vi "STANDALONE_VI.vi"() -> ()   [LabVIEW 2018]
uses:
  <vilib>/Instr/_visa.llb/VISA Open Access Mode.ctl
  <vilib>/express/express signal manip/GetorSetDDTAttributes/Shared VIs/TimeType.ctl
  <vilib>/Analysis/baseanly.llb/Mean (DBL).vi
  <vilib>/Analysis/2dsp.llb/1D Auto Correlation (DBL).vi
  <vilib>/Instr/_visa.llb/VISA Configure Serial Port (Instr).vi
  <vilib>/express/express signal manip/GetorSetDDTAttributes/Shared VIs/TimeMode Enum to Boolean.vi
  <vilib>/express/express shared/transition.llb/Dynamic To Waveform Array.vi
  <vilib>/express/express signal manip/GetorSetDDTAttributes/Set DDT Attributes/SetT0.vi
  <vilib>/express/express shared/transition.llb/Waveform Array To Dynamic.vi
  <vilib>/Analysis/2dsp.llb/1D Cross Correlation (DBL).vi
  <vilib>/express/express signal manip/GetorSetDDTAttributes/Set DDT Attributes/Set DDT Properties.xnode
  <vilib>/express/express signal manip/GetorSetDDTAttributes/Shared VIs/GetSetShared.lvlib
  <vilib>/Analysis/NI_AALPro.lvlib
  <vilib>/Analysis/NI_AALBase.lvlib
panel:
  out "DEBUG BUFFER":string
  out "Load Force (N)":dbl
  out "Grip Force (N)":dbl
  out "Calibration Complete":bool
  in  "?":bool
  out "x .or. y? 2":bool
  out "Load Force Plot":dynamicdata(graph)
  out "Grip Force Plot":dynamicdata(graph)
  out "x-y 4":u32
  out "Goniometer Angle Plot":dynamicdata(graph)
  out "Elbow Angle (deg)":dbl
  in  "Start Training\nButton":bool
  out "Calibration Timer":string caption="Elapsed Time Text"
  out "Elbow Angle Offset":dbl format="%0.2f"
  out "Grip Force at MZ":dbl format="%0.2f"
  out "Load Force at MZ":dbl format="%0.2f"
  in  "Calibrate System\nButton":bool
  in  "VISA resource name":refnum<visa-resource-name>="COM4"
  out "error out":errorcluster
  out "x*y":dbl
  out "max index(es)":i32
  out "max":dbl
  out "max value":dbl
  out "size":i32
  out "Waveform Graph":dbl[](graph)
  out "max index":i32
  out "Delay (ms)":i32
  out "GF min":dbl
  out "GF max":dbl
  out "LF min":dbl
  out "LF max":dbl
  # "SET UP"
  # "PLOTS"
  # "TRAINING SESSION"
  # "SYSTEM CALIBRATION"
  # "REAL-TIME DATA"
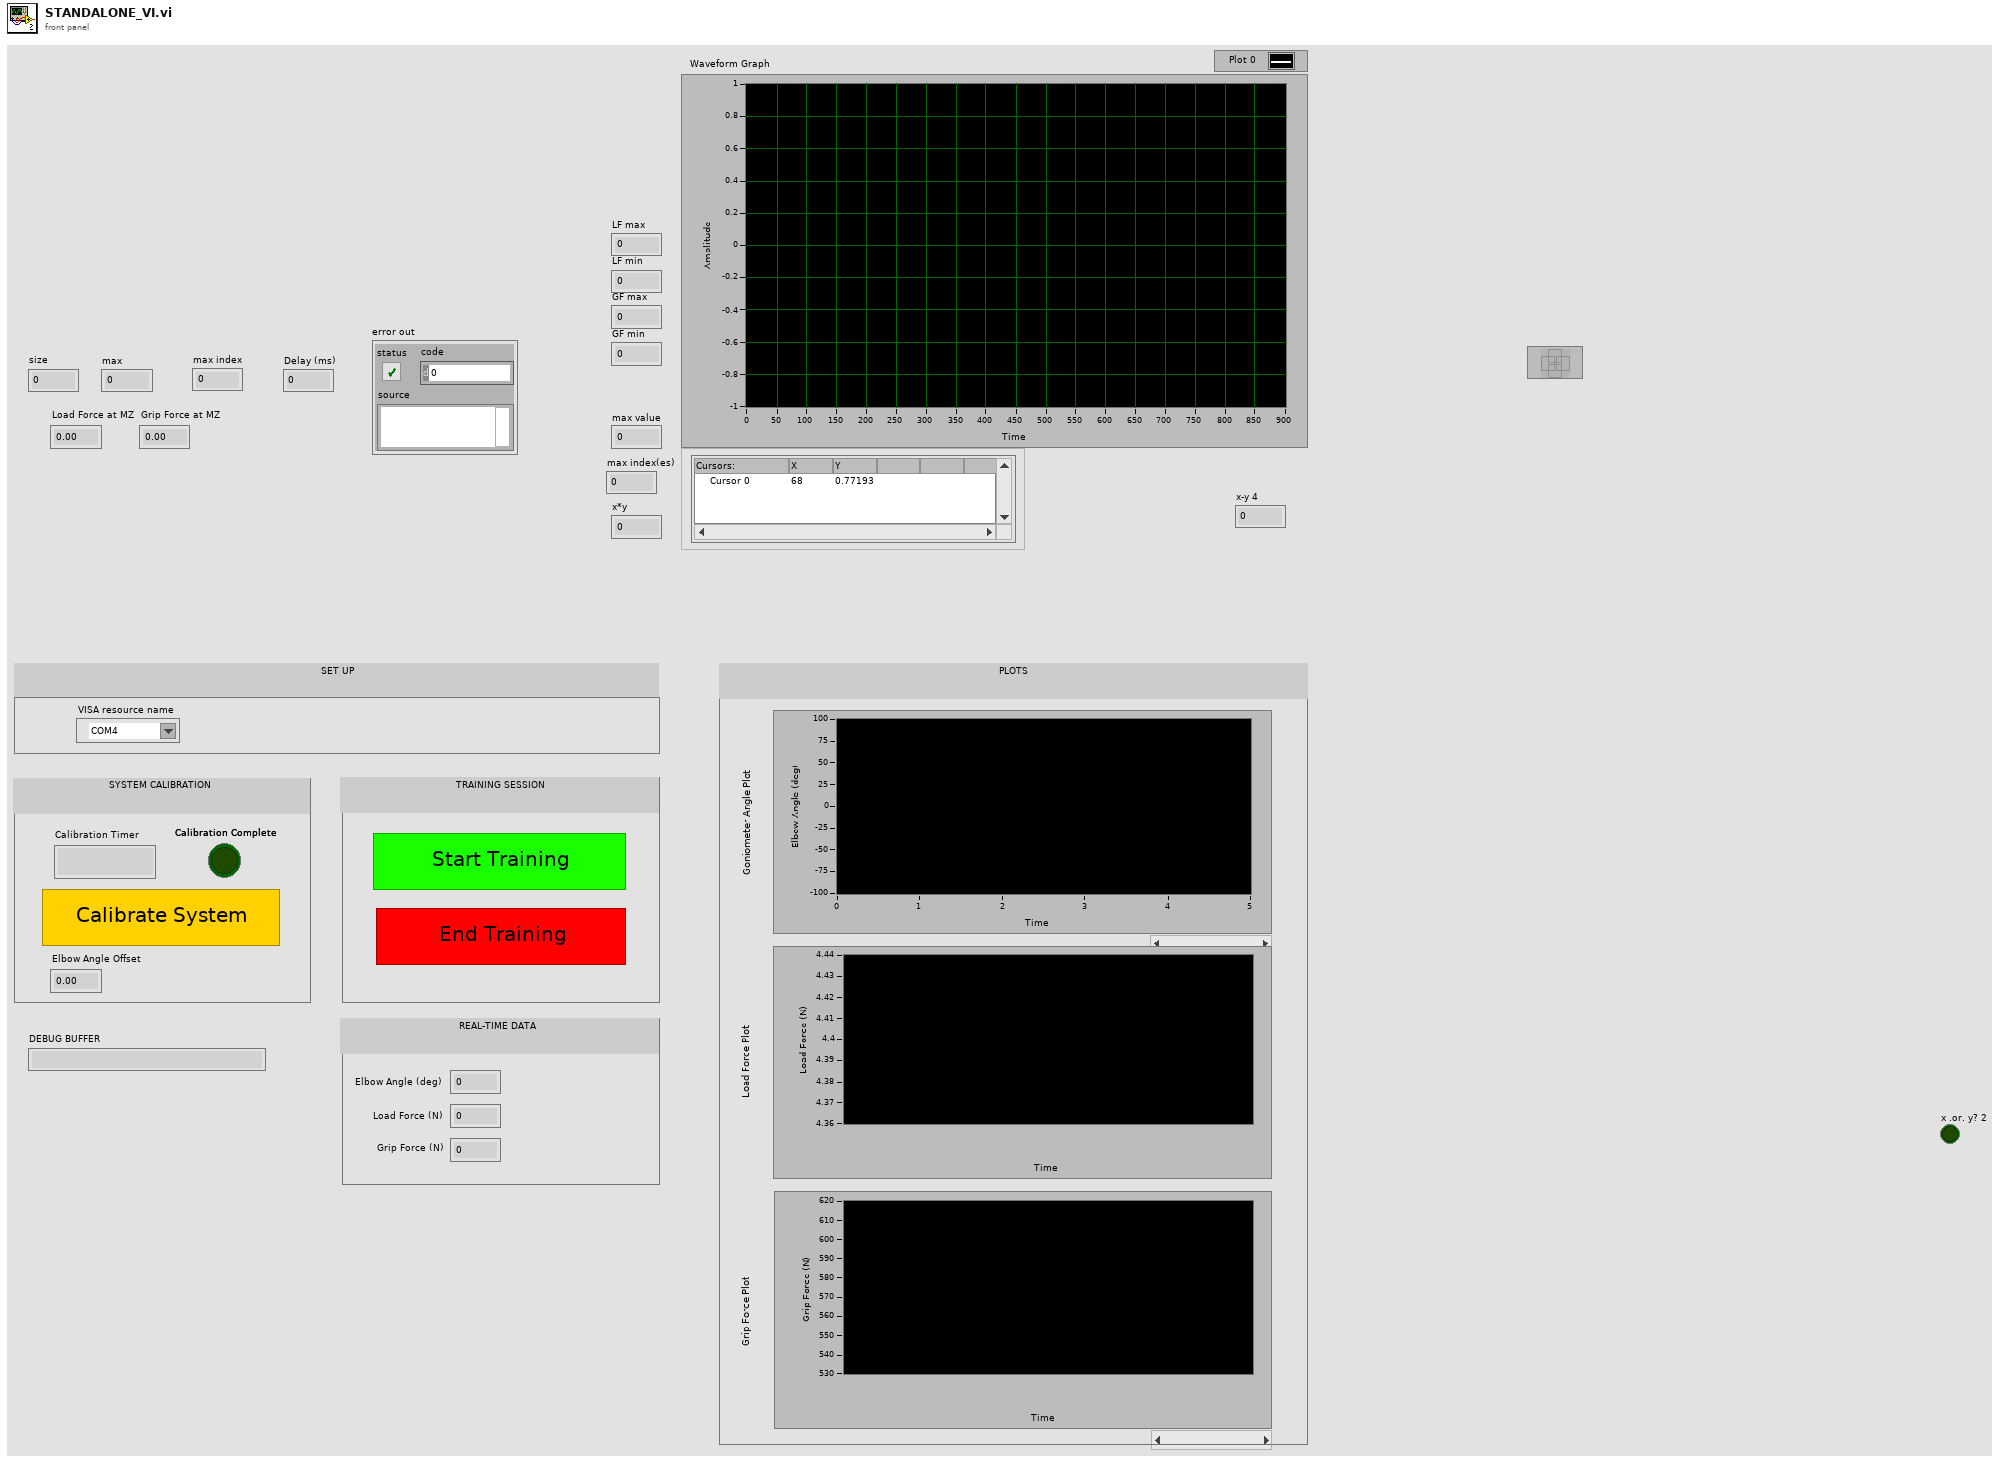
[diagram p1: front panel]
types:
  T1 = typedef "VISA Open Access Mode.ctl" = u32
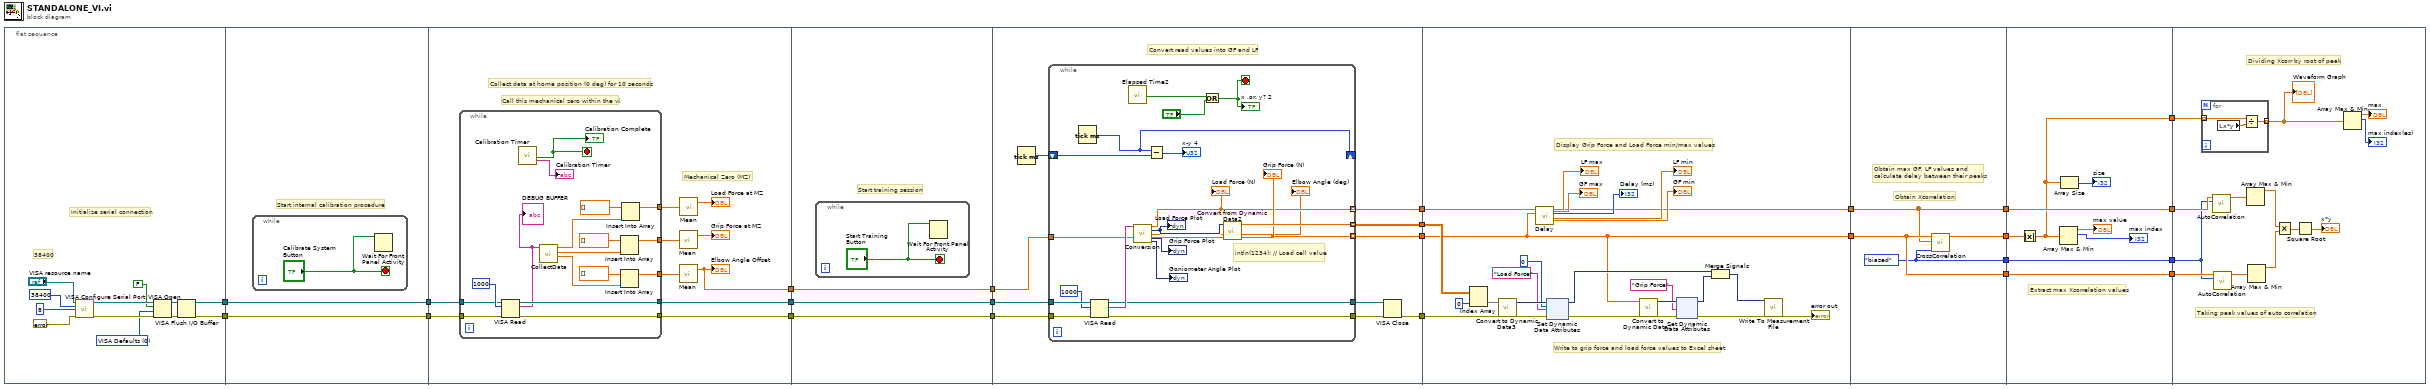
[diagram p0: block diagram]
diagram:
  n1 = flat-sequence {
    tunnel: [w28] -> w24
    tunnel: [w27] -> w23
    tunnel: [w38] -> w22
    tunnel: w24 -> [w38]
    tunnel: [w37] -> w21
    tunnel: w23 -> [w37]
    tunnel: w22 -> [w49]
    tunnel: [w46] -> w20
    tunnel: w21 -> [w48]
    tunnel: [w47] -> w19
    tunnel: [w40] -> w12
    tunnel: w20 -> [w69]
    tunnel: [w69] -> w18
    tunnel: w19 -> [w68]
    tunnel: [w68] -> w17
    tunnel: [w67] -> w13
    tunnel: w12 -> [w67]
    tunnel: w18 -> [w80]
    tunnel: w17 -> [w79]
    tunnel: [w77] -> w16
    tunnel: [w76] -> w15
    tunnel: [w75] -> w14
    tunnel: w13 -> [w74]
    tunnel: [w71] -> w11
    tunnel: w16 -> [w102]
    tunnel: w15 -> [w105]
    tunnel: w14 -> [w101]
    tunnel: w11 -> [w104]
    tunnel: [w102] -> w10
    tunnel: [w101] -> w9
    tunnel: w10 -> [w161]
    tunnel: w9 -> [w162]
    tunnel: [w163] -> w8
    tunnel: [w160] -> w7
    tunnel: [w162] -> w5
    tunnel: [w161] -> w3
    tunnel: w8 -> [w168]
    tunnel: w7 -> [w171]
    tunnel: [w171] -> w6
    tunnel: w5 -> [w170]
    tunnel: [w170] -> w4
    tunnel: w3 -> [w169]
    tunnel: [w169] -> w2
    tunnel: [w164] -> w1
    tunnel: w6 -> [w172]
    tunnel: w4 -> [w181]
    tunnel: w2 -> [w180]
    tunnel: w1 -> [w179]
    frame #0 {
      w26 = T1 0 items=["VISA Defaults"=0, "Exclusive Lock"=1, "Load Configured Settings"=4] ("Access Mode")
      # "38400"
      # "Initialize serial connection"
      n2 = call-poly "VISA Configure Serial Port"("VISA resource name"="VISA resource name", "baud rate (9600)"=u32 38400, "data bits (8)"=u16 8, "error in (no error)"=errorcluster {"status"=FALSE, "code"=0, "source"=""}) -> ("VISA resource name out"=w34:refnum<visa-resource-name>, "error out"=w32:errorcluster)  [unwired: 10 in]
      n3 = VISA Open(duplicate session (F)=FALSE, access mode=w26, error in (no error)=w32, VISA resource name=w34) -> (VISA resource name=w35:refnum<visa-resource-name>, error out=w36:errorcluster)  [unwired: 1 in]
      n4 = VISA Flush I/O Buffer(VISA resource name=w35, error in (no error)=w36) -> (VISA resource name out=w27:refnum<visa-resource-name>, error out=w28:errorcluster)  [unwired: 1 in]
    }
    frame #1 {
      # "Start internal calibration procedure"
      n5 = while {
        stop <- "Calibrate System\nButton" stop-if-true
        n6 = Wait For Front Panel Activity(3:"Calibrate System\nButton") -> ()  [unwired: 2 in, 1 out]
      }
    }
    frame #2 {
      # "Call this mechanical zero within the vi"
      # "Mechanical Zero (MZ)"
      # "Collect data at home position (0 deg) for 10 seconds"
      n7 = while {
        tunnel: w49 -> [w65]
        tunnel: w48 -> [w64]
        tunnel: [w62] -> w47
        tunnel: [w61] -> w46
        tunnel: [w60] -> w45
        tunnel: [w58] -> w44
        tunnel: [w56] -> w43
        stop <- w51 stop-if-true
        n8 = VISA Read(VISA resource name=w64, byte count=u32 1000, error in (no error)=w65) -> (VISA resource name out=w62:refnum<visa-resource-name>, read buffer=w50:string, error out=w61:errorcluster)  [unwired: 1 out]
        "DEBUG BUFFER" <- w50
        n9 = call "Calibration Timer"() -> ("Time has Elapsed"=w51:bool, "Elapsed Time Text"=→"Calibration Timer":string)  [unwired: 12 in, 6 out]
        "Calibration Complete" <- w51
        n10 = call "CollectData.vi"("read buffer"=w50) -> ("Elbow Angle"=w57:dbl, "Grip Force (GF)"=w59:dbl, "Load Force (LF)"=w63:dbl)  [unwired: 8 in]
        n11 = Insert Into Array(array=dbl[] [], new element=w59) -> (w58:dbl[])  [unwired: 1 in]
        n12 = Insert Into Array(array=dbl[] [], new element=w57) -> (w56:dbl[])  [unwired: 1 in]
        n13 = Insert Into Array(array=dbl[] [], new element=w63) -> (w60:dbl[])  [unwired: 1 in]
      }
      n14 = call-poly <vilib>:"Mean.vi"("X"=w44) -> ("mean"=→"Grip Force at MZ":dbl)  [unwired: 1 out]
      n15 = call-poly <vilib>:"Mean.vi"("X"=w43) -> ("mean"=w40:dbl)  [unwired: 1 out]
      "Elbow Angle Offset" <- w40
      n16 = call-poly <vilib>:"Mean.vi"("X"=w45) -> ("mean"=→"Load Force at MZ":dbl)  [unwired: 1 out]
    }
    frame #3 {
      # "Start training session"
      n17 = while {
        stop <- "Start Training\nButton" stop-if-true
        n18 = Wait For Front Panel Activity(3:"Start Training\nButton") -> ()  [unwired: 2 in, 1 out]
      }
    }
    frame #4 {
      # "Convert read values into GF and LF"
      n19 = Tick Count (ms)() -> (millisecond timer value=w78:u32)
      n20 = while {
        tunnel: [w100] -> w72
        tunnel: [w95] -> w73
        tunnel: [w92] -> w76 mode=indexing
        shift-right: [w91] -> _
        shift-left: w78 -> [w90]
        tunnel: [w88] -> w75 mode=indexing
        tunnel: [w87] -> w77 mode=indexing
        tunnel: w80 -> [w84]
        tunnel: w79 -> [w83]
        tunnel: w74 -> [w81]
        stop <- w97 stop-if-true
        # "intln(1234); // Load cell value"
        n21 = Tick Count (ms)() -> (millisecond timer value=w91:u32)
        n22 = VISA Read(VISA resource name=w83, byte count=u32 1000, error in (no error)=w84) -> (VISA resource name out=w95:refnum<visa-resource-name>, read buffer=w96:string, error out=w100:errorcluster)  [unwired: 1 out]
        n23 = call "Elapsed Time2"() -> ("Time has Elapsed"=w99:bool)  [unwired: 12 in, 7 out]
        n24 = call "Conversion.vi"("read buffer"=w96, "Mechanical Zero"=w81) -> ("LF"=w87:dbl, "Load Force"=w93:dynamicdata, "Elbow Angle (deg)"=→"Elbow Angle (deg)":dbl, "GF"=w88:dbl, "Grip Force"=→"Grip Force Plot":dynamicdata, "Goniometer\nAngle Raw"=→"Goniometer Angle Plot":dynamicdata)  [unwired: 8 in]
        "Load Force Plot" <- w93
        "Grip Force (N)" <- w88
        "Load Force (N)" <- w87
        n25 = Subtract(x=w91, y=w90) -> (x-y=→"x-y 4":u32)
        n26 = Or(x=w99, y="?") -> (x .or. y?=w97:bool)
        "x .or. y? 2" <- w97
        n27 = call "Convert from Dynamic Data2"("Dynamic Data Type"=w93) -> ("Array"=w92:dbl[])  [unwired: 3 in]
      }
      n28 = VISA Close(VISA resource name=w73, error in (no error)=w72) -> (error out=w71:errorcluster)
    }
    frame #5 {
      # "Display Grip Force and Load Force min/max values"
      # "Write to grip force and load force values to Excel sheet"
      n29 = Index Array(array=w105, index (col)=0 ("disabled index (col)")) -> (element=w120:dbl[])  [unwired: 1 in]
      n30 = call "Convert to Dynamic Data3"("Array"=w120) -> ("Dynamic Data Type"=w114:dynamicdata)  [unwired: 3 in]
      n31 = call "Delay.vi"("GF array"=w101, "LF array"=w102) -> ("LF min"=→"LF min":dbl, "Delay"=→"Delay (ms)":i32, "LF max"=→"LF max":dbl, "GF min"=→"GF min":dbl, "GF max"=→"GF max":dbl)  [unwired: 5 in]
      n32 = xnode "Set Dynamic\nData Attributes"("Signals In"=w114, "error in"=w104, "Signal Index"=0, "Signal Name"="Load Force") -> ("Signals Out"=w110:dynamicdata, "error out"=w109:errorcluster)  [unwired: 1 in]
      n33 = call "Convert to Dynamic Data2"("Array"=w101) -> ("Dynamic Data Type"=w121:dynamicdata)  [unwired: 3 in]
      n34 = xnode "Set Dynamic\nData Attributes"("Signals In"=w121, "error in"=w109, "Signal Name"="Grip Force") -> ("Signals Out"=w111:dynamicdata, "error out"=w113:errorcluster)  [unwired: 2 in]
      n35 = Merge Signals(w110, w111) -> (w112:dynamicdata)
      n36 = call "Write To Measurement File"("Signals"=w112, "error in (no error)"=w113) -> ("error out"=→"error out":errorcluster)  [unwired: 15 in, 2 out]
    }
    frame #6 {
      w160 = enum32{"none", "unbiased", "biased"}."biased" ("normalization")
      # "Obtain Xcorrelation"
      # "Obtain max GF, LF values and\ncalculate delay between their peaks"
      n37 = call-poly <vilib>:"CrossCorrelation.vi"("normalization"=w160, "Y"=w161, "X"=w162) -> ("Rxy"=w163:dbl[])  [unwired: 7 in, 1 out]
    }
    frame #7 {
      # "Extract max Xcorrelation values"
      n38 = Absolute Value(x=w168) -> (abs(x)=w164:dbl[])
      n39 = Array Max & Min(array=w164) -> (max value=→"max value":dbl, max index (indices)=→"max index":i32)  [unwired: 2 out]
      n40 = Array Size(array=w164) -> (size(s)=→"size":i32)
    }
    frame #8 {
      # "Taking peak values of auto correlation"
      # "Dividing Xcorr by root of peak"
      n41 = for {
        tunnel: w179 -> [w187] mode=indexing
        tunnel: [w186] -> w182 mode=indexing
        n42 = local read "x*y"() -> (w185:dbl)
        n43 = Divide(x=w187, y=w185) -> (x/y=w186:dbl)
      }
      "Waveform Graph" <- w182
      n44 = call-poly <vilib>:"AutoCorrelation.vi"("normalization"=w172, "X"=w180) -> ("Rxx"=w178:dbl[])  [unwired: 8 in, 1 out]
      n45 = call-poly <vilib>:"AutoCorrelation.vi"("normalization"=w172, "X"=w181) -> ("Rxx"=w177:dbl[])  [unwired: 8 in, 1 out]
      n46 = Array Max & Min(array=w178) -> (max value=w176:dbl)  [unwired: 3 out]
      n47 = Array Max & Min(array=w177) -> (max value=w175:dbl)  [unwired: 3 out]
      n48 = Multiply(x=w176, y=w175) -> (x*y=w174:dbl)
      n49 = Square Root(x=w174) -> (sqrt(x)=→"x*y":dbl)
      n50 = Array Max & Min(array=w182) -> (max value=→"max":dbl, max index (indices)=→"max index(es)":i32)  [unwired: 2 out]
    }
  }
